vi "openConnection.vi"(5 "Data cluster out":T1, 6 "Boolean":bool, 7 "error out 2":errorcluster) -> (0 "port":refnum<k16>, 1 "listener ID":refnum<k5>, 2 "connection ID":refnum<k16>, 3 "error out":errorcluster, 4 "Numeric":u16)   [LabVIEW 2009]
uses:
  dataCluster.ctl
  <vilib>/vision/Image Controls.llb/IMAQ Image.ctl
  DataQueueTypeDef.ctl
  <vilib>/Utility/tcp.llb/UDP Multicast Read-Only Open.vi
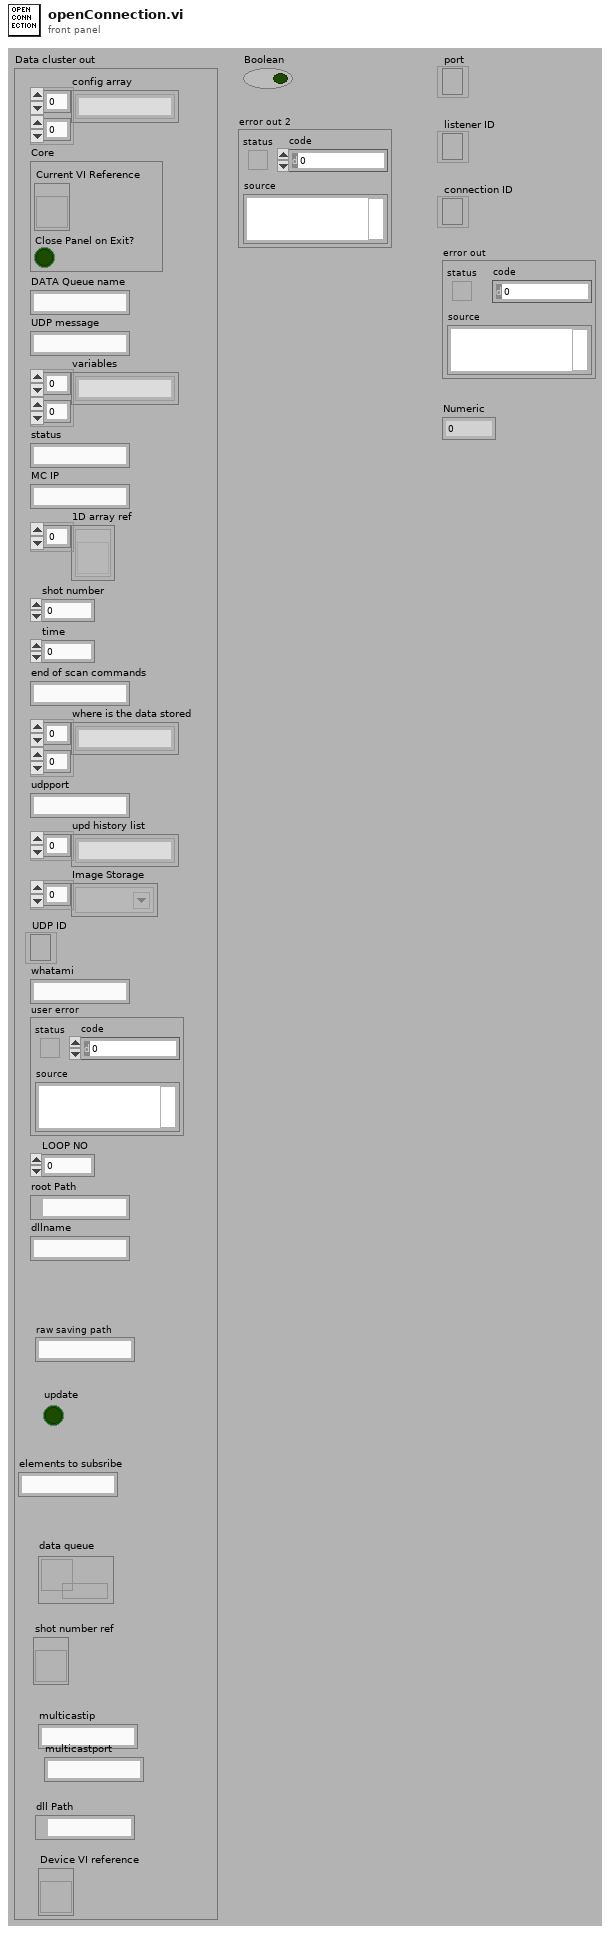
[diagram p1: front panel]
types:
  T1 = typedef "dataCluster.ctl" = cluster{"config array":string[][], "Core":cluster{"Current VI Reference":refnum<vi>, "Close Panel on Exit?":bool}, "DATA Queue name":string, "UDP message":string, "variables":string[][], "status":string, "MC IP":string, "1D array ref":refnum<vi>[], "shot number":i32, "time":u32, "end of scan commands":string, "where is the data stored":string[][], "udpport":string, "upd history list":string[], "Image Storage":T2[], "UDP ID":refnum<k16>, "whatami":string, "user error":errorcluster, "LOOP NO":u32, "root Path":path, "dllname":string, "raw saving path":string, "update":bool, "elements to subsribe":string, "data queue":refnum<queue>, "shot number ref":refnum<vi>, "multicastip":string, "multicastport":string, "dll Path":path, "Device VI reference":refnum<vi>}
  T2 = typedef "IMAQ Image.ctl" = refnum<image>
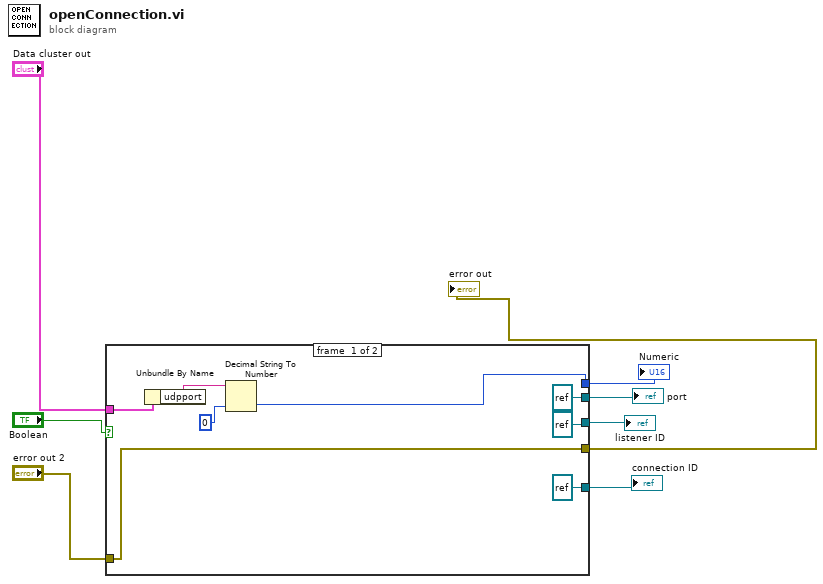
[diagram p0: block diagram]
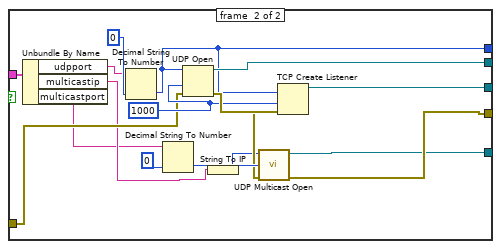
[diagram p2: hidden frame]
diagram:
  n1 = case shown="True" "Boolean" {
    tunnel: "Data cluster out" -> [w12 w31]
    tunnel: "error out 2" -> [w16 w27]
    tunnel: [w16 w25] -> w3
    tunnel: [refnum<k16> refnum ("port") w20] -> w5
    tunnel: [refnum<k5> refnum ("listener ID") w19] -> w6
    tunnel: [refnum<k16> refnum ("connection ID") w18] -> w7
    tunnel: [w9 w17] -> w8
    frame #0 {
      n2 = Unbundle By Name(w12) -> ("udpport"=w11:string)
      n3 = Decimal String To Number(string=w11, default (0L)=u16 0 ("default (0 I32)")) -> (number=w9:u16)  [unwired: 1 in, 1 out]
    }
    frame #1 {
      w28 = 1000 ("timeout ms (25000)")
      n4 = Unbundle By Name(w31) -> ("udpport"=w32:string, "multicastip"=w24:string, "multicastport"=w23:string)
      n5 = Decimal String To Number(string=w32, default (0L)=u16 0 ("default (0 I32)")) -> (number=w17:u16)  [unwired: 1 in, 1 out]
      n6 = Decimal String To Number(string=w23, default (0L)=u16 0 ("port")) -> (number=w22:u16)  [unwired: 1 in, 1 out]
      n7 = UDP Open(8:w27, 9:w28, 11:w17) -> (port=w20:refnum<k16>, 0:w30:errorcluster)  [unwired: 2 in, 1 out]
      n8 = String To IP(1:w24) -> (0:w29:u32)
      n9 = TCP Create Listener(8:w30, 9:w28, 10:w17) -> (0:w26:errorcluster, 3:w19:refnum<k5>)  [unwired: 2 in, 1 out]
      n10 = call-poly <vilib>:"UDP Multicast Open.vi"("error in (no error)"=w26, "multicast addr"=w29, "port"=w22) -> ("error out"=w25:errorcluster, "connection ID"=w18:refnum<k16>)  [unwired: 1 in, 6 out]
    }
  }
  "Numeric" <- w8
  "connection ID" <- w7
  "listener ID" <- w6
  "port" <- w5
  "error out" <- w3
